vi "Do.vi"(8 "error in (no error)":errorcluster, 10 "Actor in":refnum<class "Actor.lvclass">, 11 "Conceret HVAC System Tiles Info Msg in":refnum<class "Conceret HVAC System Tiles Info Msg.lvclass">) -> (0 "error out":errorcluster, 2 "Actor out":refnum<class "Actor.lvclass">)   [LabVIEW 2013, in "HVAC System View.lvlib" / "Conceret HVAC System Tiles Info Msg.lvclass"]
doc: "(<B>Filename</B>: Actor Framework.lvlib:Message.lvclass:Do.vi)\n\nDefines what a message does when it is received by an actor. Generally, a message instructs an actor to invoke one of its methods.\n\nBy default, this method does nothing. A child class must override it to define behavior. Create a child class by using the Actor Framework Message Maker dialog box."
uses:
  Conceret HVAC System Tiles Info Msg.lvclass
  <vilib>/ActorFramework/Actor/Actor.lvclass
  HVAC System View/HVAC System View.lvclass
  Models/HVAC System Model Messages/Abstract HVAC System Tiles Info Msg/Abstract HVAC System Tiles Info Msg.lvclass
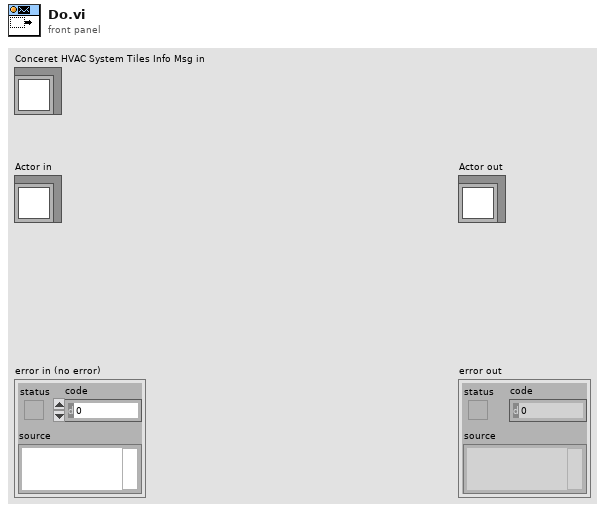
[diagram p1: front panel]
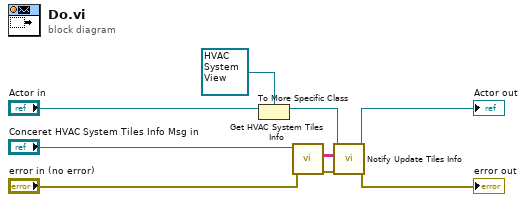
[diagram p0: block diagram]
diagram:
  n1 = To More Specific Class(target class=refnum<class "HVAC System View.lvclass"> refnum ("HVAC System View.lvlib:HVAC System View.lvclass"), reference="Actor in") -> (specific class reference=w6:refnum<class "HVAC System View.lvclass">)  [unwired: 1 in, 1 out]
  n2 = call "Get HVAC System Tiles Info.vi"("error in (no error)"="error in (no error)", "Abstract HVAC System Tiles Info Msg in"="Conceret HVAC System Tiles Info Msg in") -> ("error out"=w5:errorcluster, "HVAC System Tiles Info"=w1:string[][])  [unwired: 7 in, 1 out]
  n3 = call "Notify Update Tiles Info.vi"("error in (no error)"=w5, "HVAC System Tiles Info"=w1, "Test Channel View in"=w6) -> ("error out"=→"error out":errorcluster, "Test Channel View out"=→"Actor out":refnum<class "HVAC System View.lvclass">)  [unwired: 7 in]
